vi "Connect.vi"(8 "error in":errorcluster, 9 "timeout ms (1000)":i32=1000, 10 "Address":string, 11 "RawSocket Handler in":refnum<class "RawSocket TCP Handler.lvclass">) -> (0 "error out":errorcluster, 3 "RawSocket Handler out":refnum<class "RawSocket TCP Handler.lvclass">)   [LabVIEW 2020, in "wamplv.lvlib" / "RawSocket TCP Handler.lvclass"]
uses:
  RawSocket TCP Handler.lvclass
  C:/local/wamplv/Private/Comm Handlers/CommHandlerBase/CommHandlerBase.lvclass
  C:/local/wamplv/Private/Comm Handlers/TCPSocketBasedCommHandlerBase/TCPSocketBasedCommHandlerBase.lvclass
  <vilib>/LabVIEW Open Source Project/OpenURI/uri/URI.lvclass/URI.ctl
  RawSocket TCP Handler.lvclass/RawSocket TCP Handler.ctl
  <vilib>/LabVIEW Open Source Project/OpenURI/uri/URI.lvclass
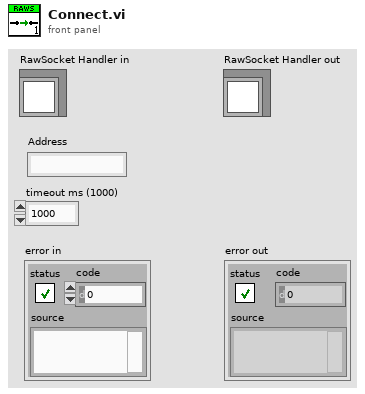
[diagram p1: front panel]
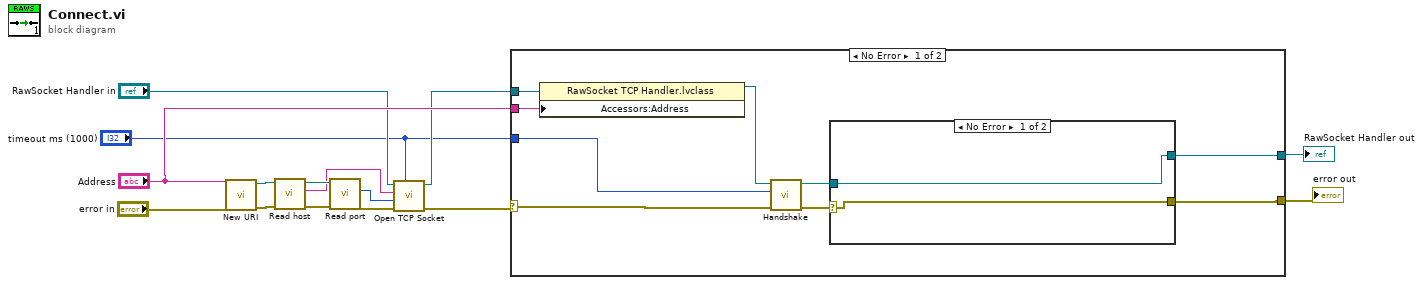
[diagram p0: block diagram]
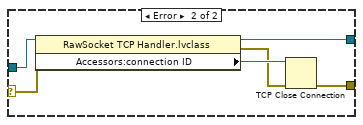
[diagram p2: hidden frame]
diagram:
  n1 = call <vilib>:"New URI.vi"("error in (no error)"="error in", "URI"="Address") -> ("error out"=w13:errorcluster, "URI"=w14:refnum<class "URI.lvclass">)  [unwired: 8 in]
  n2 = call <vilib>:"Read host.vi"("error in (no error)"=w13, "URI in"=w14) -> ("error out"=w12:errorcluster, "host"=w7:string, "URI out"=w11:refnum<class "URI.lvclass">)  [unwired: 7 in]
  n3 = call <vilib>:"Read port.vi"("error in (no error)"=w12, "URI in"=w11) -> ("error out"=w5:errorcluster, "port"=w6:u16)  [unwired: 7 in, 1 out]
  n4 = call-dynamic "Open TCP Socket.vi"("timeout ms (60000)"="timeout ms (1000)", "error in (no error)"=w5, "remote port or service name"=w6, "address"=w7, "TCPSocketBasedCommHandlerBase in"="RawSocket Handler in") -> ("error out"=w2:errorcluster, "TCPSocketBasedCommHandlerBase out"=w3:refnum<class "RawSocket TCP Handler.lvclass">)  [unwired: 4 in, 1 out]
  n5 = case shown="No Error" w2 {
    selector: w2 -> [w17 w34]
    tunnel: w3 -> [w24 w33]
    tunnel: "Address" -> [w23 _]
    tunnel: [w20 w34] -> w9
    tunnel: [w18 w33] -> w8
    tunnel: "timeout ms (1000)" -> [w16 _]
    frame No Error {
      n6 = property class="RawSocket TCP Handler.lvclass"(reference=w24, "Accessors:Address"=w23) -> (reference out=w22:refnum<class "RawSocket TCP Handler.lvclass">)  [unwired: 1 in, 1 out]
      n7 = call "Handshake.vi"("error in"=w17, "timeout ms (25000)"=w16, "RawSocket Handler in"=w22) -> ("error out"=w21:errorcluster, "RawSocket Handler out"=w19:refnum<class "RawSocket TCP Handler.lvclass">)  [unwired: 7 in]
      n8 = case shown="No Error" w21 {
        selector: w21 -> [w26 w29]
        tunnel: [w26 w32] -> w20
        tunnel: w19 -> [w25 w31]
        tunnel: [w25 w27] -> w18
        frame No Error {
        }
        frame Error {
          n9 = property class="RawSocket TCP Handler.lvclass"(reference=w31, error in=w29) -> (reference out=w27:refnum<class "RawSocket TCP Handler.lvclass">, error out=w28:errorcluster, "Accessors:connection ID"=w30:refnum<k5>)
          n10 = TCP Close Connection(connection ID=w30, error in (no error)=w28) -> (error out=w32:errorcluster)  [unwired: 1 in, 1 out]
        }
      }
    }
    frame Error {
    }
  }
  "RawSocket Handler out" <- w8
  "error out" <- w9
